vi "_Update Serial DAC.vi"(4 "Wait(12Ticks)":u8=12, 5 "DIN (F)":bool, 6 "FSYNCH (T)":bool=TRUE, 7 "Clock (F)":bool) -> ()   [LabVIEW 2012]
uses:
  <vilib>/eio/EIONode/EIONode.xnode
  Instance           1 26Saved   _Update Serial DAC .vi
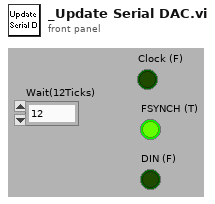
[diagram p1: front panel]
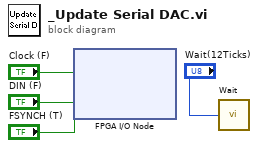
[diagram p0: block diagram]
diagram:
  n1 = xnode "FPGA I/O Node"("Port1/DIO0"="Clock (F)", "Port0/DIO8"="DIN (F)", "Port1/DIO2"="FSYNCH (T)") -> ()  [unwired: 3 in, 3 out]
  n2 = call "Wait"("Count(Ticks)"="Wait(12Ticks)") -> ()  [unwired: 1 out]
